vi "CLD 13 Flow Rate Calculations.vi"(8 "Fehler (Eingang)":T1, 11 "Cluster (Eingang)":T2) -> (0 "Fehler (Ausgang)":T1, 3 "Cluster (Ausgang)":T2)   [LabVIEW 2009]
doc: "CLD 13 - Logik zur Änderung der Flussrate. Mit dem Algorithmus wird die Flussrate in Einer-Schritten herabgesetzt, bis sie null erreicht. Dadurch wird die Funktion zur Berechnung der verstrichenen Zeit vereinfacht."
uses:
  CLD 13 Data Cluster.ctl
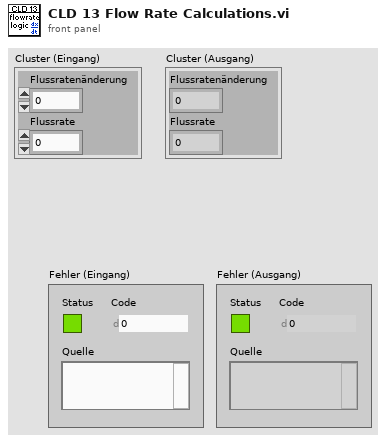
[diagram p1: front panel]
types:
  T1 = cluster{"Status":bool, "Code":i32, "Quelle":string}
  T2 = typedef "CLD 13 Data Cluster.ctl" = cluster{"Flussratenänderung":i8, "Flussrate":i8}
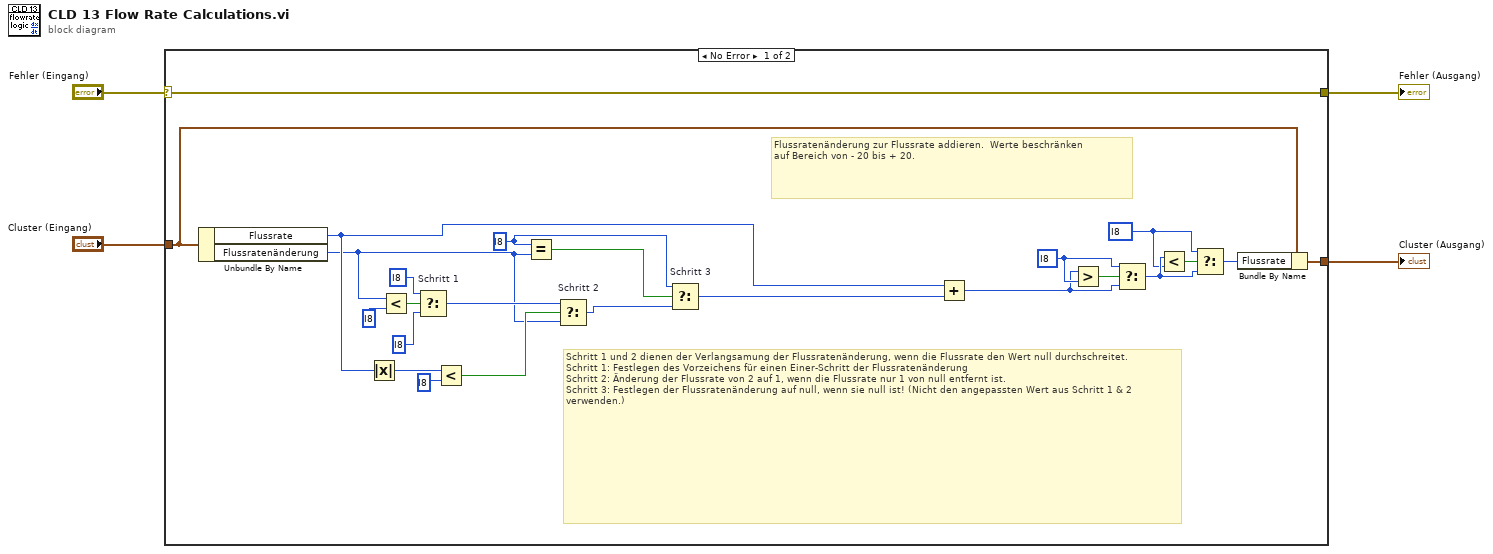
[diagram p0: block diagram]
diagram:
  n1 = case shown="No Error" "Fehler (Eingang)" {
    selector: "Fehler (Eingang)" -> [w5 w30]
    tunnel: [w20 w29] -> w4
    tunnel: "Cluster (Eingang)" -> [w18 w29]
    tunnel: [w5 w30] -> w1
    frame #0 {
      w27 = i8 ? ("x")
      w16 = i8 ? ("y")
      w14 = i8 ? ("y")
      # "Flussratenänderung zur Flussrate addieren.  Werte beschränken \nauf Bereich von - 20 bis + 20."
      # "Schritt 1 und 2 dienen der Verlangsamung der Flussratenänderung, wenn die Flussrate den Wert null durchschreitet.\nSchritt 1: Festlegen des Vorzeichens für einen Einer-Schritt der Flussratenänderung \nSchritt 2: Änderung der Flussrate von 2 auf 1, wenn die Flussrate nur 1 von null entfernt ist.\nSchritt 3: Festlegen der Flussratenänderung auf null, wenn sie null ist! (Nicht den angepassten Wert aus Schritt 1 & 2 verwenden.)"
      n2 = Unbundle By Name(w18) -> ("Flussrate"=w8:i8, "Flussratenänderung"=w7:i8)
      n3 = Absolute Value(x=w8) -> (abs(x)=w10:i8)
      n4 = Less?(x=w7, y=i8 ? ("x")) -> (x < y?=w22:bool)
      n5 = Select "Schritt 1"(t=i8 ?, s=w22, f=i8 ? ("t")) -> (s? t:f=w25:i8)
      n6 = Less?(x=w10, y=i8 ?) -> (x < y?=w11:bool)
      n7 = Equal?(x=w27, y=w7) -> (x = y?=w26:bool)
      n8 = Select "Schritt 2"(t=w25, s=w11, f=w7) -> (s? t:f=w28:i8)
      n9 = Select "Schritt 3"(t=w27, s=w26, f=w28) -> (s? t:f=w6:i8)
      n10 = Add(x=w8, y=w6) -> (x+y=w13:i8)
      n11 = Greater?(x=w13, y=w14) -> (0:w12:bool)
      n12 = Select(t=w14, s=w12, f=w13) -> (s? t:f=w17:i8)
      n13 = Less?(x=w17, y=w16) -> (x < y?=w15:bool)
      n14 = Select(t=w16, s=w15, f=w17) -> (s? t:f=w19:i8)
      n15 = Bundle By Name(cluster=w18, "Flussrate"=w19) -> (w20:T2)
    }
    frame #1 {
    }
  }
  "Cluster (Ausgang)" <- w4
  "Fehler (Ausgang)" <- w1
